vi "Constants.vi"() -> ()   [LabVIEW 2026, in "Nominal Core Streaming Shared.lvlib"]
doc: "Use this Global VI to access the GUIDs assigned to the page resources of the Custom Device."
uses:
  Nominal Core Streaming Shared.lvlib
panel:
  in  "Tab Control":enum32{"GUIDs", "Constants", "Properties"}(tab)
  in  "GUID.Decimation":string="d4c1a460-d7a8-41fc-a423-153e611c0c5c"
  in  "GUID.Time Channel":string="dd2615b5-9b09-4bc9-afd6-539be4c59745"
  in  "Stream":string="58b2bb4a-3d23-4307-a360-2df60781b45b"
  in  "Dataset":string="103cdb43-9024-4ccf-befa-0c5cd138060c"
  in  "GUID.Status":string="b79b0641-9f91-4c5b-82f7-02598dffe8d5"
  in  "GUID.Enable":string="4a38a077-dc8d-46d0-821c-69c63979c629"
  in  "Nominal Core Streaming":string="936fc33f-b1a6-49ce-bce7-e773e6cb4405"
  in  "stream.buffer size":string="stream_buffer_size"
  in  "stream.nominal url":string="stream_base_url"
  in  "time.convert type":string="time_convert_type"
  in  "stream.api key":string="stream_api_key"
  in  "Time Channel Name":string="Time source"
  in  "status channel name":string="Status"
  in  "Decimation channel name":string="Decimation"
  in  "enable channel name":string="Enable"
  in  "stream.dataset id":string="stream_dataset_id"
  in  "stream.dataset name":string="stream_dataset_name"
  in  "stream.asset id":string="stream_asset_id"
  in  "stream.identifier selection":string="stream_identifier_selection"
  in  "Compiled.Settings":string="Compiled.Settings"
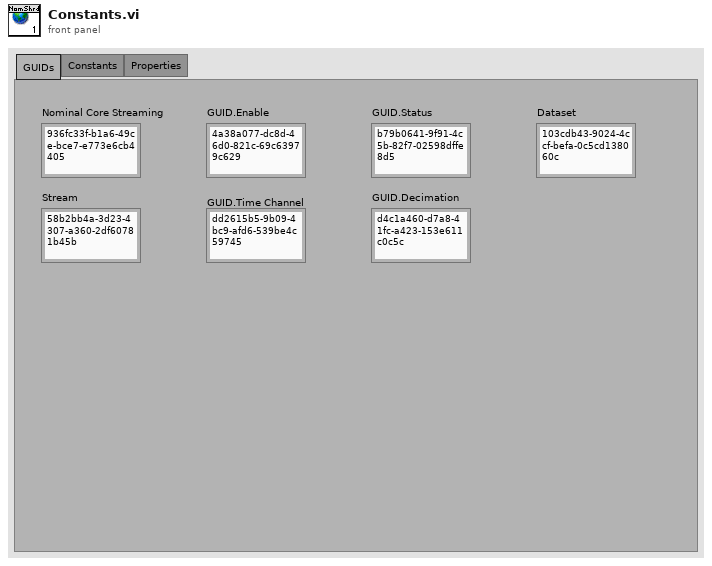
[diagram p1: front panel]
diagram:
